vi "fgt get pressure Status.vi"(8 "error in (no error)":errorcluster, 11 "pressureIndex":u32) -> (0 "error out":errorcluster)   [LabVIEW 2016, in "fgt_SDK.lvlib"]
doc: "Get detailed information of pressure channel status. \nThis function is meant to be invoked after calling a pressure related function which returns an error code.\nRetrieved information of last error contains controller position and a string detail."
uses:
  fgt_SDK.lvlib
  TypeDefs/fgt_STATUS_INFO.ctl
  TypeDefs/fgt_INSTRUMENT_TYPE.ctl
  dlls/fgt_SDK_32.dll
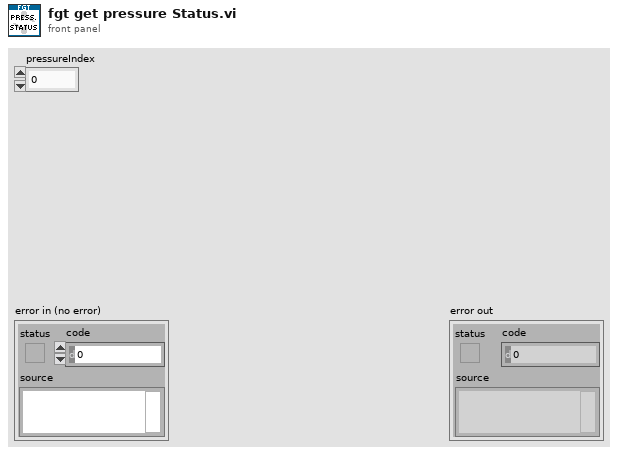
[diagram p1: front panel]
types:
  T1 = typedef "fgt_SDK.lvlib/fgt_STATUS_INFO.ctl" = cluster{"InstrType":T2, "instrSN":u16, "errorCode":u8, "infoCode":u8, "detail":string}
  T2 = typedef "fgt_SDK.lvlib/fgt_INSTRUMENT_TYPE.ctl" = enum32{"None", "MFCS", "MFCS_EZ", "FRP", "LineUP", "IPS", "ESS", "F_OEM", "CFU", "NIFS"}
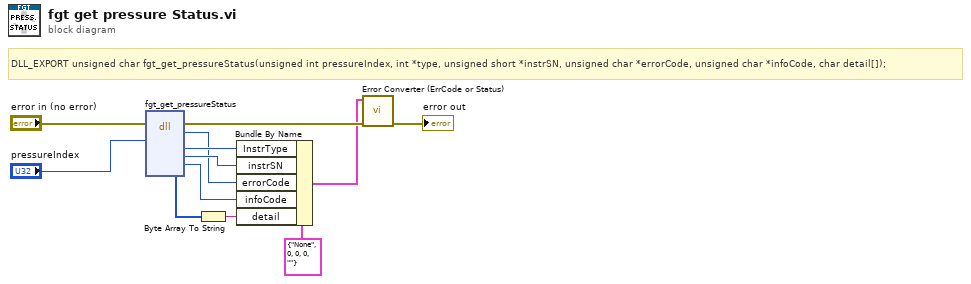
[diagram p0: block diagram]
diagram:
  # "DLL_EXPORT unsigned char fgt_get_pressureStatus(unsigned int pressureIndex, int *type, unsigned short *instrSN, unsigned char *errorCode, unsigned char *infoCode, char detail[]);"
  n1 = dll-call lib="C:/projects/SDK/fgt-sdk-labview/dlls/fgt_SDK_*.*" fn="fgt_get_pressureStatus"(error in="error in (no error)", "pressureIndex"="pressureIndex") -> (error out=w10:errorcluster, "return type"=w3:u8, "type"=w7:i32, "instrSN"=w6:u16, "infoCode"=w5:u8, "detail"=w2:i8[])  [unwired: 7 in, 1 out]
  n2 = Byte Array To String(unsigned byte array=w2) -> (string=w1:string)
  n3 = Bundle By Name(cluster=T1 {"InstrType"=enum."None", "instrSN"=0, "errorCode"=0, "infoCode"=0, "detail"=""} ("Cluster"), "InstrType"=w7, "instrSN"=w6, "errorCode"=w3, "infoCode"=w5, "detail"=w1) -> (w4:T1)
  n4 = call "Error Converter (ErrCode or Status).vi"("error in (no error)"=w10, "StatusInfo"=w4) -> ("error out"=→"error out":errorcluster)  [unwired: 9 in]
